vi "Open PV Connections.vi"(1 "URLs":string[](array[string]), 3 "Access (R/W allowed)":T1, 4 "Error In":errorcluster) -> (0 "PV Connections":refnum<class "PVConnection.lvclass">[](array[class]), 2 "Error Out":errorcluster)   [LabVIEW 2015, in "CS++ProcessVariables.lvlib"]
doc: "Open references to process variables."
uses:
  CS++ProcessVariables.lvlib
  PVConnection/PVConnection.lvclass
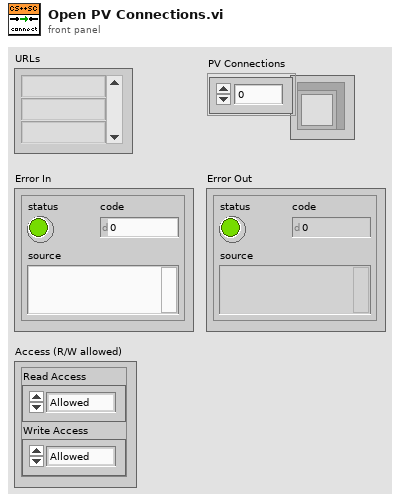
[diagram p1: front panel]
types:
  T1 = cluster{"Read Access":enum8{"Allowed", "Required", "None"}, "Write Access":enum8{"Allowed", "Required", "None"}}
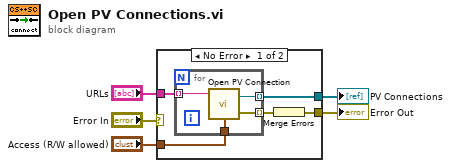
[diagram p0: block diagram]
diagram:
  n1 = case shown="No Error" "Error In" {
    selector: "Error In" -> [_ w15]
    tunnel: "URLs" -> [w10 _]
    tunnel: [w9 _] -> w4
    tunnel: [w7 w15] -> w3
    tunnel: "Access (R/W allowed)" -> [w6 _]
    frame No Error {
      n2 = for {
        tunnel: w10 -> [w14] mode=indexing
        tunnel: w6 -> [w11]
        tunnel: [w13] -> w9 mode=indexing
        tunnel: [w12] -> w8 mode=indexing
        n3 = call "Open PV Connection.vi"("PV URL"=w14, "Access (R/W allowed)"=w11) -> ("PVConnection"=w13:refnum<class "PVConnection.lvclass">, "Error Out"=w12:errorcluster)  [unwired: 1 in]
      }
      n4 = Merge Errors(w8) -> (w7:errorcluster)
    }
    frame Error {
    }
  }
  "PV Connections" <- w4
  "Error Out" <- w3
